vi "Read VISA.vi"(8 "error in (no error)":errorcluster, 10 "VISA Refnum in":refnum<visa-resource-name>, 11 "Serial Device in":refnum<class "Serial Device.lvclass">) -> (0 "error out":errorcluster, 1 "Serial Response":string, 2 "VISA resource name out":refnum<visa-resource-name>, 3 "Serial Device out":refnum<class "Serial Device.lvclass">)   [LabVIEW 2020, in "Serial Device.lvclass"]
uses:
  Serial Device.lvclass
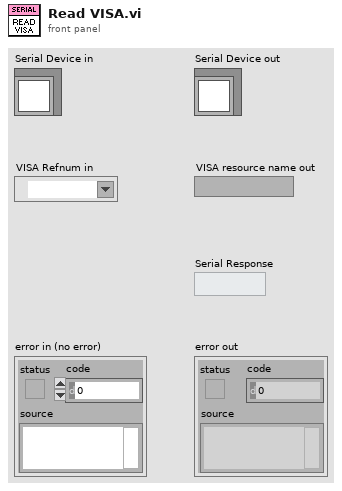
[diagram p1: front panel]
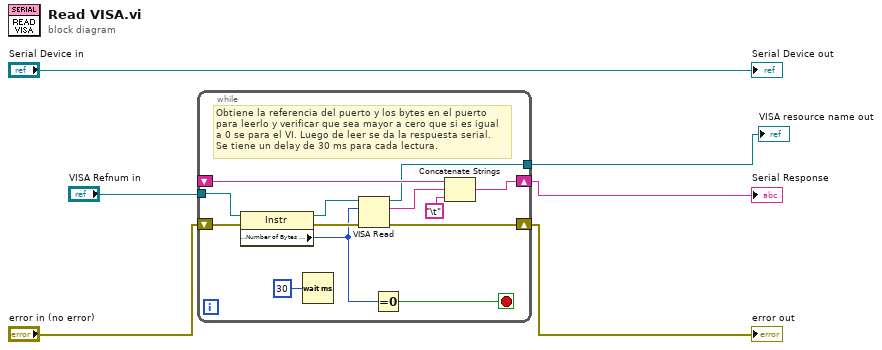
[diagram p0: block diagram]
diagram:
  n1 = while {
    tunnel: "VISA Refnum in" -> [w19]
    shift-right: [w18] -> w3
    shift-left: "error in (no error)" -> [w17]
    shift-right: [w13] -> w1
    shift-left: _ -> [w14]
    tunnel: [w9] -> w2
    stop <- w10 stop-if-true
    # "Obtiene la referencia del puerto y los bytes en el puerto\npara leerlo y verificar que sea mayor a cero que si es igual\na 0 se para el VI. Luego de leer se da la respuesta serial.\nSe tiene un delay de 30 ms para cada lectura."
    n2 = property class="Instr"(reference=w19, error in=w17) -> (reference out=w15:refnum<visa-resource-name>, error out=w16:errorcluster, "Serial Settings:Number of Bytes at Serial Port"=w11:u32)
    n3 = Wait (ms)(milliseconds to wait=u32 30) -> ()  [unwired: 1 out]
    n4 = VISA Read(VISA resource name=w15, byte count=w11, error in (no error)=w16) -> (VISA resource name out=w9:refnum<visa-resource-name>, read buffer=w8:string, error out=w18:errorcluster)  [unwired: 1 out]
    n5 = Equal To 0?(x=w11) -> (x = 0?=w10:bool)
    n6 = Concatenate Strings(w14, w8, "\t") -> (w13:string)
  }
  "error out" <- w3
  "Serial Response" <- w1
  "VISA resource name out" <- w2
  "Serial Device out" <- "Serial Device in"
